vi "Find Custom Device by Name.vi"(8 "error in":errorcluster, 10 "custom device name":string, 11 "target":refnum<k24>) -> (0 "error out":errorcluster, 2 "custom device":T1 format="%.0x", 3 "target out":refnum<k24>, 4 "found?":bool)   [LabVIEW 2020, in "AIM MIL-STD-1553 Scripting.lvlib"]
doc: "Within the specified <b>target</b>, this VI searches for an AIM MIL-STD 1553 Custom Device with the specified <b>custom device name</b> and returns a reference to the <b>custom device</b>."
uses:
  AIM MIL-STD-1553 Scripting.lvlib
  NationalInstruments.VeriStand.SystemDefinitionAPI
  <vilib>/NI VeriStand/Custom Device API/Custom Device Item Ref.ctl
  Constants.vi
  <vilib>/NI VeriStand/Custom Device API/Custom Device API.lvlib
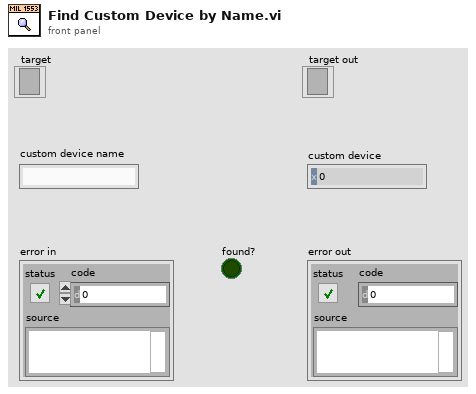
[diagram p1: front panel]
types:
  T1 = typedef "Custom Device API.lvlib/Custom Device Item Ref.ctl" = u64
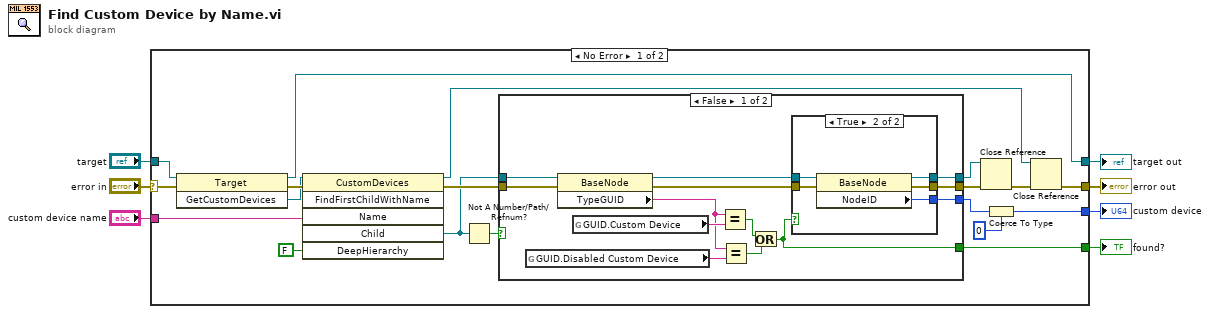
[diagram p0: block diagram]
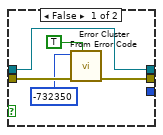
[diagram p2: hidden frame]
diagram:
  n1 = case shown="No Error" "error in" {
    selector: "error in" -> [w21 w53]
    tunnel: "target" -> [w22 w52]
    tunnel: [w16 w53] -> w5
    tunnel: [w9 _] -> w2
    tunnel: [w18 w52] -> w4
    tunnel: "custom device name" -> [w15 _]
    tunnel: [w11 _] -> w1
    frame No Error {
      n2 = invoke on="Invoke Node" class="Target" method="GetCustomDevices"(reference=w22, error in=w21) -> (reference out=w18:refnum<k24>, error out=w26:errorcluster, "GetCustomDevices"=w25:refnum<k24>)  [unwired: 1 in]
      n3 = invoke on="Invoke Node" class="CustomDevices" method="FindFirstChildWithName"(reference=w25, error in=w26, "Name"=w15, "DeepHierarchy"=FALSE) -> (reference out=w19:refnum<k24>, error out=w17:errorcluster, "Child"=w14:refnum<k24>)  [unwired: 2 in, 3 out]
      n4 = Not A Number/Path/Refnum?(number/path/refnum=w14) -> (NaN/Path/Refnum?=w13:bool)
      n5 = case shown="False" w13 {
        tunnel: [w39 w50] -> w24
        tunnel: [w38 w51] -> w23
        tunnel: w17 -> [w36 w51]
        tunnel: w14 -> [w35 w50]
        tunnel: [w37 _] -> w10
        tunnel: [w27 _] -> w11
        frame False {
          n6 = global read "Constants.vi" "GUID.Disabled Custom Device"() -> (w31:string)
          n7 = property on="Property Node" class="BaseNode"(reference=w35, error in=w36) -> (reference out=w32:refnum<k24>, error out=w33:errorcluster, "TypeGUID"=w30:string)
          n8 = global read "Constants.vi" "GUID.Custom Device"() -> (w34:string)
          n9 = Equal?(x=w30, y=w34) -> (x = y?=w29:bool)
          n10 = Equal?(x=w30, y=w31) -> (x = y?=w28:bool)
          n11 = Or(x=w29, y=w28) -> (x .or. y?=w27:bool)
          n12 = case shown="True" w27 {
            tunnel: [w41 w46] -> w38
            tunnel: w33 -> [w43 w48]
            tunnel: w32 -> [w44 w49]
            tunnel: [w44 w47] -> w39
            tunnel: [_ w45] -> w37
            frame False {
              n13 = call <vilib>:"Error Cluster From Error Code.vi"("show call chain? (False)"=TRUE, "error in (no error)"=w43, "error code (0)"=-732350) -> ("error out"=w41:errorcluster)  [unwired: 6 in]
            }
            frame True {
              n14 = property on="Property Node" class="BaseNode"(reference=w49, error in=w48) -> (reference out=w47:refnum<k24>, error out=w46:errorcluster, "NodeID"=w45:u64)
            }
          }
        }
        frame True {
        }
      }
      n15 = Close Reference(reference=w24, error in (no error)=w23) -> (error out=w20:errorcluster)
      n16 = Coerce To Type(0:w10, 1:T1 0 ("Ballard MIL-STD 1553 custom device")) -> (2:w9:T1)
      n17 = Close Reference(reference=w19, error in (no error)=w20) -> (error out=w16:errorcluster)
    }
    frame Error {
    }
  }
  "error out" <- w5
  "target out" <- w4
  "custom device" <- w2
  "found?" <- w1
